vi "StartData.vi"(8 "error in (no error)":errorcluster, 11 "Class In":refnum<class "C37.118 Sim.lvclass">) -> (0 "error out":errorcluster, 3 "Class Out":refnum<class "C37.118 Sim.lvclass">)   [LabVIEW 2018, in "SensorPlugins.lvlib" / "C37.118 Sim.lvclass"]
uses:
  C37.118 Sim.lvclass
  C:/projects/ICDAS/NistPluggableModules/Sensor/SensorPlugins/PmuBaseClass/PmuBase.lvclass
  PmuBaseClass/PmuBase.lvclass/PmuBase.ctl
  C37.118 Sim.lvclass/C37.118 Sim.ctl
  PmuBaseClass/Accessors/Read PmuConfig.vi
  Accessors/Read Function.vi
  PmuBaseClass/Accessors/Write PmuConfig.vi
  Accessors/Write Function.vi
  FGen/MemberClasses/FunctionBaseClass/FunctionBase.lvclass
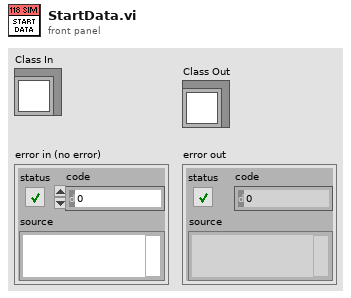
[diagram p1: front panel]
types:
  T1 = typedef "SensorPlugins.lvlib/PmuBase.lvclass/PmuConfig.ctl" = cluster{"Class":enum16{"M", "P"}, "Fs":i32, "F0":i32, "FSamp":i32, "SettlingTime":dbl, "T0":ext}
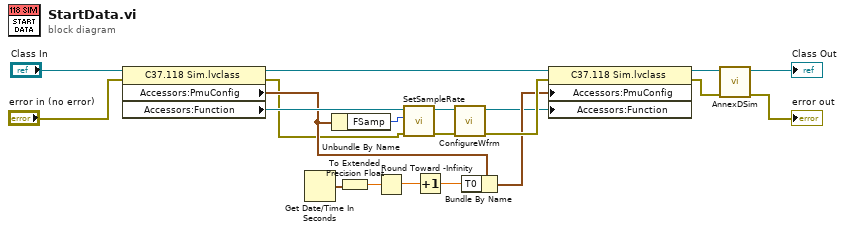
[diagram p0: block diagram]
diagram:
  n1 = property class="C37.118 Sim.lvclass"(reference="Class In", error in="error in (no error)") -> (reference out=w18:refnum<class "C37.118 Sim.lvclass">, error out=w4:errorcluster, "Accessors:PmuConfig"=w6:T1, "Accessors:Function"=w7:refnum<class "FunctionBase.lvclass">)
  n2 = Get Date/Time In Seconds() -> (seconds since 1Jan1904=w12:timestamp)
  n3 = Unbundle By Name(w6) -> ("FSamp"=w5:i32)
  n4 = To Extended Precision Float(1:w12) -> (0:w11:ext)
  n5 = Round Toward -Infinity(1:w11) -> (0:w10:ext)
  n6 = call-dynamic "SetSampleRate.vi"("error in (no error)"=w4, "SampleRate"=w5, "FunctionBase in"=w7) -> ("error out"=w2:errorcluster, "FunctionBase out"=w3:refnum<class "FunctionBase.lvclass">)  [unwired: 7 in]
  n7 = Increment(x=w10) -> (x+1=w9:ext)
  n8 = call-dynamic "ConfigureWfrm.vi"("error in (no error)"=w2, "FunctionBase in"=w3) -> ("error out"=w13:errorcluster, "FunctionBase out"=w1:refnum<class "FunctionBase.lvclass">)  [unwired: 8 in]
  n9 = Bundle By Name(cluster=w6, "T0"=w9) -> (w8:T1)
  n10 = property class="C37.118 Sim.lvclass"(reference=w18, error in=w13, "Accessors:PmuConfig"=w8, "Accessors:Function"=w1) -> (reference out=w17:refnum<class "C37.118 Sim.lvclass">, error out=w15:errorcluster)
  n11 = call "AnnexDSim.vi"("error in (no error)"=w15, "C37.118 Sim in"=w17) -> ("error out"=→"error out":errorcluster, "C37.118 Sim out"=→"Class Out":refnum<class "C37.118 Sim.lvclass">)  [unwired: 8 in]
